vi "Trigger_Coincidence_Logic.vi"(9 "Peak_ch4":dbl, 10 "Peak_ch3":dbl, 11 "Peak_ch2":dbl) -> (3 "Filter-out":bool)   [LabVIEW 2019]
uses:
  SiPM_Tests_Global_Var.vi
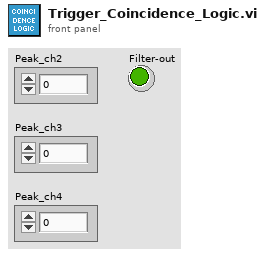
[diagram p1: front panel]
types:
  T1 = enum16{"Coincidence", "Anti-Coincidence", "Don't Care"}
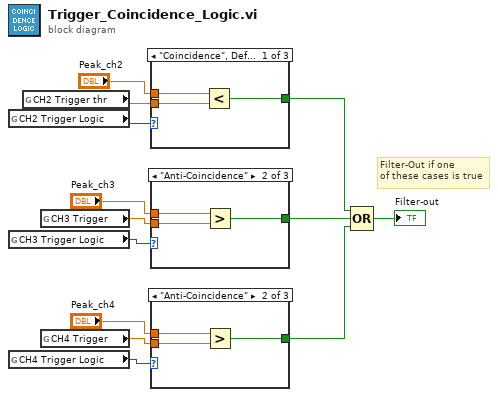
[diagram p0: block diagram]
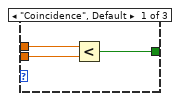
[diagram p2: hidden frame]
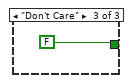
[diagram p3: hidden frame]
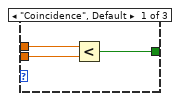
[diagram p4: hidden frame]
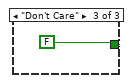
[diagram p5: hidden frame]
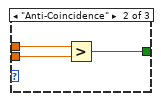
[diagram p6: hidden frame]
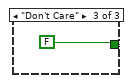
[diagram p7: hidden frame]
diagram:
  # "Filter-Out if one \nof these cases is true"
  n1 = global read "SiPM_Tests_Global_Var.vi" "CH2 Trigger Logic"() -> (w1:T1)
  n2 = global read "SiPM_Tests_Global_Var.vi" "CH3 Trigger Logic"() -> (w5:T1)
  n3 = global read "SiPM_Tests_Global_Var.vi" "CH4 Trigger Logic"() -> (w8:T1)
  n4 = global read "SiPM_Tests_Global_Var.vi" "CH2 Trigger thr"() -> (w2:dbl)
  n5 = global read "SiPM_Tests_Global_Var.vi" "CH3 Trigger"() -> (w4:dbl)
  n6 = global read "SiPM_Tests_Global_Var.vi" "CH4 Trigger"() -> (w9:dbl)
  n7 = case shown="\"Coincidence\", Default" w1 {
    tunnel: [w14 w17 FALSE] -> w10
    tunnel: w2 -> [w16 w18 _]
    tunnel: "Peak_ch2" -> [w15 w19 _]
    frame "Coincidence", Default {
      n8 = Less?(x=w15, y=w16) -> (x < y?=w14:bool)
    }
    frame "Anti-Coincidence" {
      n9 = Greater?(x=w19, y=w18) -> (0:w17:bool)
    }
    frame "Don't Care" {
    }
  }
  n10 = case shown="\"Anti-Coincidence\"" w5 {
    tunnel: [w21 w24 FALSE] -> w11
    tunnel: w4 -> [w23 w25 _]
    tunnel: "Peak_ch3" -> [w22 w26 _]
    frame "Coincidence", Default {
      n11 = Less?(x=w22, y=w23) -> (x < y?=w21:bool)
    }
    frame "Anti-Coincidence" {
      n12 = Greater?(x=w26, y=w25) -> (0:w24:bool)
    }
    frame "Don't Care" {
    }
  }
  n13 = case shown="\"Anti-Coincidence\"" w8 {
    tunnel: [w28 w31 FALSE] -> w12
    tunnel: w9 -> [w30 w32 _]
    tunnel: "Peak_ch4" -> [w29 w33 _]
    frame "Coincidence", Default {
      n14 = Less?(x=w29, y=w30) -> (x < y?=w28:bool)
    }
    frame "Anti-Coincidence" {
      n15 = Greater?(x=w33, y=w32) -> (0:w31:bool)
    }
    frame "Don't Care" {
    }
  }
  n16 = Compound Arithmetic op=OR(w10, w11, w12) -> (→"Filter-out":bool)
